vi "Enums.vi"(8 "Array Of Clusters":T1(array[cluster])=[{"Numeros"=enum."Uno", "Array"=[enum."un", enum."trois"]}], 9 "Array":T2[](array[typedef])=[enum."Value 22", enum."Value 44", enum."Foo", enum."Value 11", enum."Bar"], 10 "Cluster":cluster{"Numeric":dbl, "Enum":T2}={"Numeric"=1111.0, "Enum"=enum."Value 33"}, 11 "Enum":enum16{"aaaa", "bbbb", "cccc", "dddd"}(ring)=enum."cccc") -> ()   [LabVIEW 2010]
uses:
  EnumControl.ctl
panel:
  in  "stop":bool
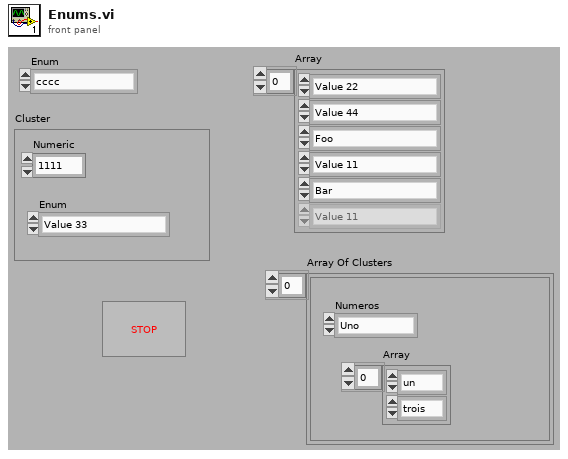
[diagram p1: front panel]
types:
  T1 = cluster{"Numeros":enum16{"Cero", "Uno", "Dos", "Tres"}, "Array":enum16{"zéro", "un", "deux", "trois"}[]}[]
  T2 = typedef "EnumControl.ctl" = enum16{"Value 11", "Value 22", "Foo", "Value 33", "Bar", "Value 44"}
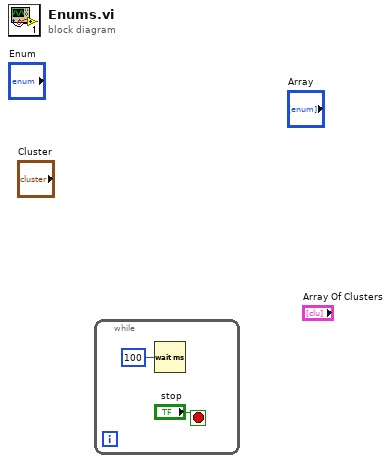
[diagram p0: block diagram]
diagram:
  n1 = while {
    stop <- "stop" stop-if-true
    n2 = Wait (ms)(milliseconds to wait=u32 100) -> ()  [unwired: 1 out]
  }
